vi "Update OK State.vi"(11 "XML Export Path":path) -> (3 "OK State":T1(ring))   [LabVIEW 2014, in "SLSC configuration System Explorer.lvlib"]
uses:
  SLSC configuration System Explorer.lvlib
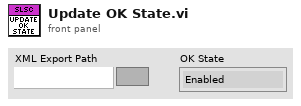
[diagram p1: front panel]
types:
  T1 = enum8{"Enabled", "Disabled", "Disabled and Grayed Out"}
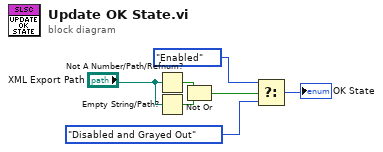
[diagram p0: block diagram]
diagram:
  n1 = Not A Number/Path/Refnum?(number/path/refnum="XML Export Path") -> (NaN/Path/Refnum?=w2:bool)
  n2 = Empty String/Path?(string/path="XML Export Path") -> (empty?=w1:bool)
  n3 = Not Or(1:w1, 2:w2) -> (0:w5:bool)
  n4 = Select(t=T1."Enabled" ("Disabled"), s=w5, f=T1."Disabled and Grayed Out" ("Disabled")) -> (s? t:f=→"OK State":T1)
